vi "LFTOF.vi"(9 "LF DOA":u32[][](array[numeric]), 10 "Col":i32, 11 "Row":i32) -> (3 "LF TOF":bool[][](array[boolean]))   [LabVIEW 2013]
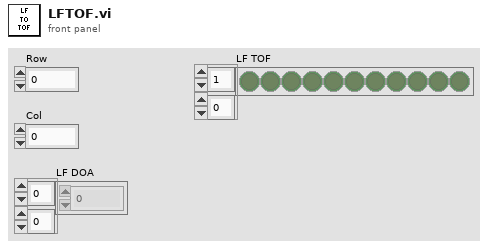
[diagram p1: front panel]
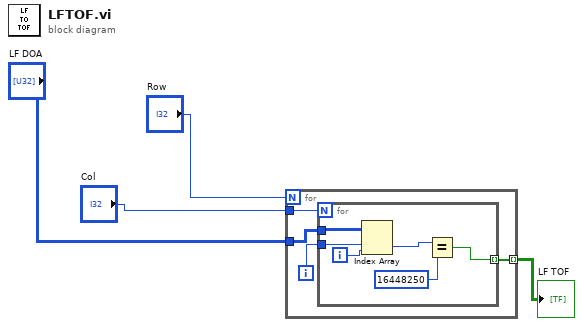
[diagram p0: block diagram]
diagram:
  n1 = for {
    N: "Row" -> [_]
    tunnel: "Col" -> [w8]
    tunnel: "LF DOA" -> [w7]
    tunnel: [w5] -> w4 mode=indexing
    i -> [w6]
    n2 = for {
      N: w8 -> [_]
      tunnel: w7 -> [w14]
      tunnel: w6 -> [w13]
      tunnel: [w9] -> w5 mode=indexing
      i -> [w12]
      n3 = Index Array(array=w14, index (row)=w13, index (col)=w12) -> (element=w11:u32)
      n4 = Equal?(x=w11, y=u32 16448250) -> (x = y?=w9:bool)
    }
  }
  "LF TOF" <- w4
